vi "ArdnoDilutionComputeRemainingTime.vi"(8 "Calib Feed Cycles":u8, 9 "Calib Mix Cycles":u16, 10 "Dilution Step":i32, 11 "Acquisition Time":u32) -> (3 "Remaining Time":dbl)   [LabVIEW 2018]
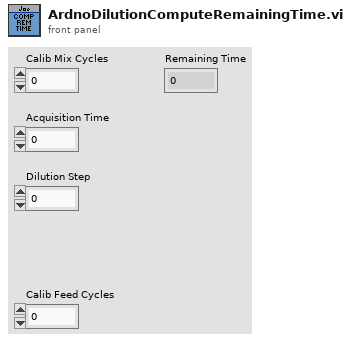
[diagram p1: front panel]
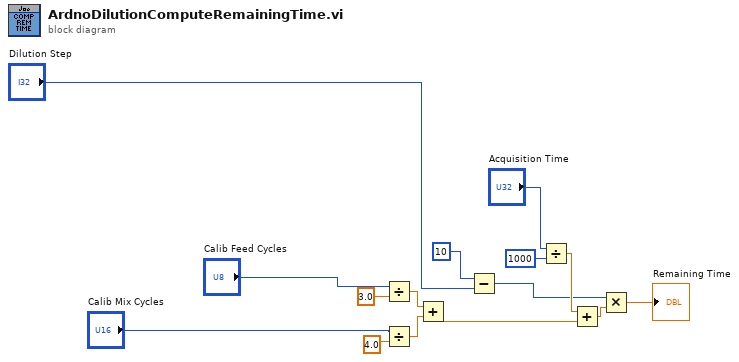
[diagram p0: block diagram]
diagram:
  n1 = Divide(x="Calib Feed Cycles", y=3.0) -> (x/y=w10:dbl)
  n2 = Divide(x="Calib Mix Cycles", y=4.0 ("Hz")) -> (x/y=w9:dbl)
  n3 = Add(x=w10, y=w9) -> (x+y=w13:dbl)
  n4 = Subtract(x=10, y="Dilution Step") -> (x-y=w6:i32)
  n5 = Divide(x="Acquisition Time", y=u32 1000) -> (x/y=w14:dbl)
  n6 = Add(x=w14, y=w13) -> (x+y=w8:dbl)
  n7 = Multiply(x=w6, y=w8) -> (x*y=→"Remaining Time":dbl)
